vi "HandleMessage.vi"(8 "error in (no error)":errorcluster, 10 "Msg":string, 11 "SHIFTER DATA":T1) -> (0 "error out":errorcluster, 3 "New BP?":bool=TRUE)   [LabVIEW 2013, in "main.lvlib"]
uses:
  main.lvlib
  Components/TypeDef - SHIFTER.ctl
  Components/Dependencies.llb/Exit Event Ref.ctl
  New Design/Controls/Reference Cluster.ctl
  MessageStructure.ctl
  Controls/Enum Variables.ctl
  Controls/Enum Save Action Events.ctl
  Components/Dependencies.llb/TLB_Dependencies.lvlib
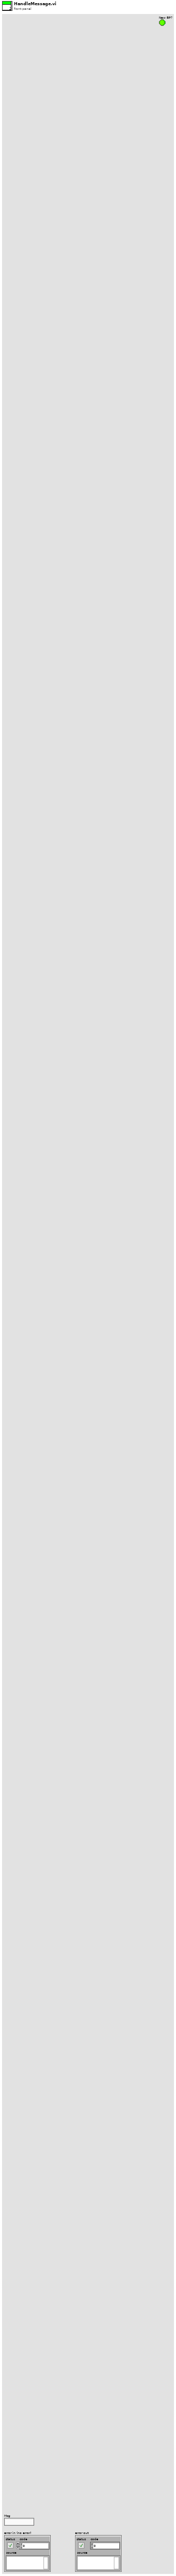
[diagram p1: front panel]
types:
  T1 = typedef "main.lvlib/TypeDef - SHIFTER.ctl" = cluster{"Exit Event":T2, "Terminate Error":errorcluster, "User Parameter Controls":refnum<vi>[], "User Parameters":cluster{"Name":string, "CPR Number":string, "Measuring Type ":string, "Measuring Technique":string, "Measuring Limb":string, "Operator":string, "Doctor":string, "Comment":string, "AdditionalInfo":string, "RightArm":string[][], "LeftArm":string[][], "PalpationRight":string, "PalpationLeft":string, "Puls":dbl, "Temp One":dbl, "Temp Two":dbl, "ActivityBox":bool}, "System Parameters":cluster{"Paper Running?":bool, "GraphSelection":bool, "Date":string, "Active Page":string}, "Data Acquisition":cluster{"Acquisition":bool, "DAQmx Task":refnum<k21>, "DAQmx Error":errorcluster, "Record number":dbl, "RecordPath":path, "AcqDataRef":refnum<vi>, "Duration":timestamp, "Queue":refnum<queue>, "Control?":bool, "RelativeRecordPath":path}, "Reference signal":cluster{"DAQmx  Task ":refnum<k21>, "Monitor":bool, "Events":dbl, "Time":timestamp, "NullEvents":dbl, "RefDataRef":refnum<vi>, "Queue":refnum<queue>}, "Data Process":cluster{"SubpanelRef":refnum<vi>, "ActiveItemTag":string, "Queue":refnum<queue>}, "System Parameter Controls":refnum<vi>[], "Database":cluster{"PatientdataRef":refnum<file>, "PatientdataPath":path, "Blue Pressure":dbl, "Red Pressure":dbl, "ActiveItemTag":string, "Height Adjustment":dbl, "BluePositionArray":dbl[][], "RedPositionArray":dbl[][], "JournalPath":path}, "MWL":cluster{"PatientID":string, "Name":string, "DICOM Info":path, "DICOM Variables":string[], "Worklist":string[][]}, "Control":cluster{"Queue":refnum<queue>, "SignalCluster":cluster{"Pump":bool, "Finger":bool, "Ankle":bool, "Fast Def":bool, "Slow Def":bool, "Init Cal":bool, "Table Pres":bool, "Table":bool}}, "PageMenu":cluster{"VI Reference":refnum<vi>, "Queue":refnum<queue>}, "Profile":cluster{"VI Reference":refnum<vi>, "Queue":refnum<queue>}, "Configuration":cluster{"VI Reference":refnum<vi>, "Queue":refnum<queue>}, "Acquisition":cluster{"VI Reference":refnum<vi>, "Queue":refnum<queue>}, "Data":cluster{"VI Reference":refnum<vi>, "Queue":refnum<queue>}, "Journal":cluster{"VI Reference":refnum<vi>, "Queue":refnum<queue>}, "cRef":T3, "Bluetooth":cluster{"Queue":refnum<queue>, "VI Reference":refnum<vi>}}
  T2 = typedef "main.lvlib/TLB_Dependencies.lvlib/Exit Event Ref.ctl" = refnum<user-event>
  T3 = typedef "main.lvlib/Reference Cluster.ctl" = cluster{"Menu":cluster{"References":cluster{"Stop Acq":refnum<vi>, "MenuExit":refnum<vi>, "MenuStartADC":refnum<vi>, "PersonalInfoString":refnum<vi>, "Profile":refnum<vi>, "Configuration":refnum<vi>, "Acquisition":refnum<vi>, "Data":refnum<vi>, "Journal":refnum<vi>}}, "Profile":cluster{"References":cluster{"Search Patient ID":refnum<vi>, "Name":refnum<vi>, "CommentStr":refnum<vi>, "Listbox Patient ID":refnum<vi>, "ListboxDoctor":refnum<vi>, "ListboxOperator":refnum<vi>, "HospitalName":refnum<vi>, "HospitalDepartment":refnum<vi>, "HospitalAddress":refnum<vi>, "EditHospInfo":refnum<vi>, "Add Patient ID Btn":refnum<vi>, "Query Worklist":refnum<vi>}}, "Configuration":cluster{"References":cluster{"ListboxMeasurementArea":refnum<vi>, "ListboxMeasurementTechnique":refnum<vi>, "ListboxMeasurementMeth":refnum<vi>, "ListboxRightSegmentNr":refnum<vi>, "ListboxLeftSegmentNr":refnum<vi>, "HeightAdjustmentInt":refnum<vi>, "PalpationRight":refnum<vi>, "PalpationLeft":refnum<vi>, "ActivityBox":refnum<vi>}, "New method":cluster{"AddNewMeasurementBtn":refnum<vi>, "Left Time Table":refnum<vi>, "Right Time Table":refnum<vi>}, "Old method":cluster{"LeftArmPressureTable":refnum<vi>, "RightArmPressureTable":refnum<vi>, "SaveArmPressureBtn":refnum<vi>, "Puls":refnum<vi>, "TempTwo":refnum<vi>, "TempOne":refnum<vi>}, "Method":string}, "Acquisition":cluster{"References":cluster{"SegmentAcqString":refnum<vi>, "RingActGraph":refnum<vi>}}, "Data":cluster{"References":cluster{"cmString":refnum<vi>, "AdjustedHeight":refnum<vi>, "Menu":refnum<vi>, "Tangent On/Off":refnum<vi>, "FilterControl":refnum<vi>}}, "Journal":cluster{"References":cluster{"ReportSelection":refnum<vi>, "Data":refnum<vi>, "GenerateReport":refnum<vi>, "Menu":refnum<vi>, "Send To PACS":refnum<vi>}}}
  T4 = typedef "main.lvlib/MessageStructure.ctl" = cluster{"Type":i32, "Device type":i32, "Date":string, "Time":string, "Serial Number":string, "Sys":i32, "Dia":i32, "Puls":i32, "MAP":i32, "Code":string}
  T5 = cluster{"Serial Number":string, "Side":string, "Ignore?":bool}
  T6 = typedef "main.lvlib/Enum Save Action Events.ctl" = enum16{"LoadReportPath", "SaveReportPath", "Load Graph Path", "Save Graph Path", "LoadDataPath", "SaveDataPath", "Load Template Path", "Save Template Path", "Load PressureFactor", "Save PressureFactor", "Init", "Load Listbox", "Save Listbox", "LoadHospInfo", "SaveHospInfo", "Load DICOM Activation", "Save DICOM Activation", "LoadDICOMInfoWL", "SaveDICOMInfoWL", "LoadDICOMInfoPACS", "SaveDICOMInfoPACS", "Load ArmCalcMethod", "Save ArmCalcMethod", "LoadItemTags", "SaveItemTags", "LoadDICOMEncoding", "SaveDICOMEncoding", "LoadJournalType", "SaveJournalType", "LoadAcqFilterType", "SaveAcqFilterType", "Load Sequence", "Save Sequence", "Load Acquisition Mode", "Save Acquisition Mode", "Load General Settings", "Save General Settings", "Load Language", "Save Language", "Load Dicom Tags", "Save Dicom Tags", "Load BT Serial", "Save BT Serial", "Load BT License", "Save BT License"}
  T7 = typedef "main.lvlib/Enum Variables.ctl" = enum16{"SetAcqFilter", "GetAcqFilter", "Set Filter", "Get Filter", "Set Height", "Get Height", "Set Recorded Height", "Get Recorded Height", "Set Blue Pressure", "Get Blue Pressure", "Set Red Pressure", "Get Red Pressure", "Init", "Reset Pressure", "Set Red Cursors", "Get Red Cursors", "Set Blue Cursors", "Get Blue Cursors", "Set Language", "Get Language", "Set Active Graphs", "Get ActiveGraphs", "Set Method", "Get Method", "Set Encryption", "Get Encryption", "Set ExcelVersion", "Get ExcelVersion", "Set DICOM Avail", "Get DICOM Avail", "Set DICOM Encode", "Get DICOM Encode", "Set JournalExport", "Get JournalExport", "Set Sequence", "Get Sequence", "Set DAQ Connected", "Get DAQ Connected", "Set Current Graph", "Get Current Graph", "Set General Settings", "Get Hyphenation", "Set Arm Calc Method", "Get Arm Calc Method", "Set Dicom Tags", "Get Dicom Tags", "Set BT Serial", "Get BT Serial", "Set BT Accepted Serials", "Get BT Accepted Serials", "Get BT License", "Set BT License"}
  T8 = cluster{"Serial Number":string, "Side":string, "Ignore?":bool}[]
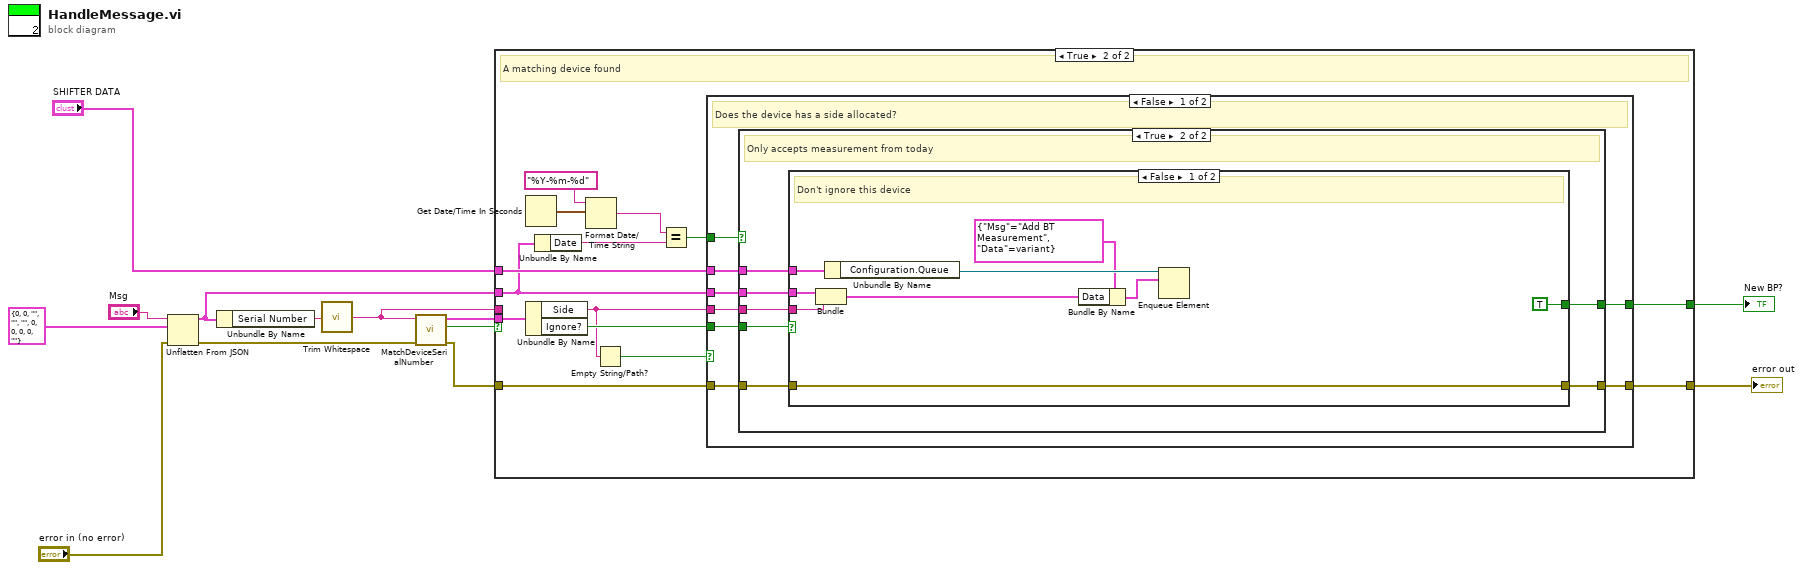
[diagram p0: block diagram]
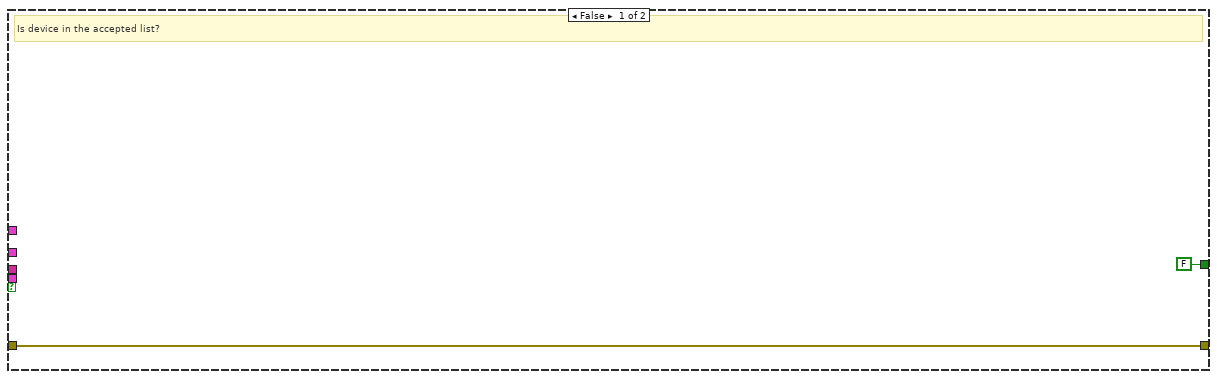
[diagram p2: hidden frame]
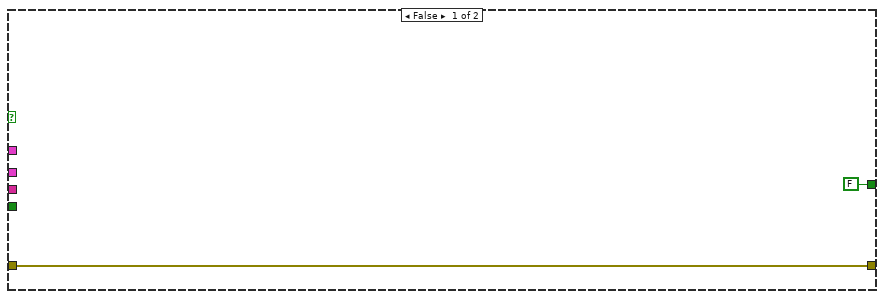
[diagram p3: hidden frame]
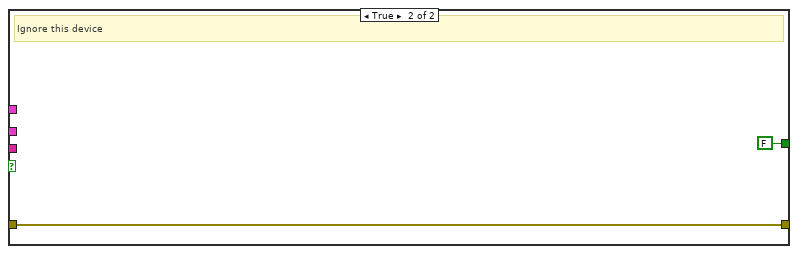
[diagram p4: hidden frame]
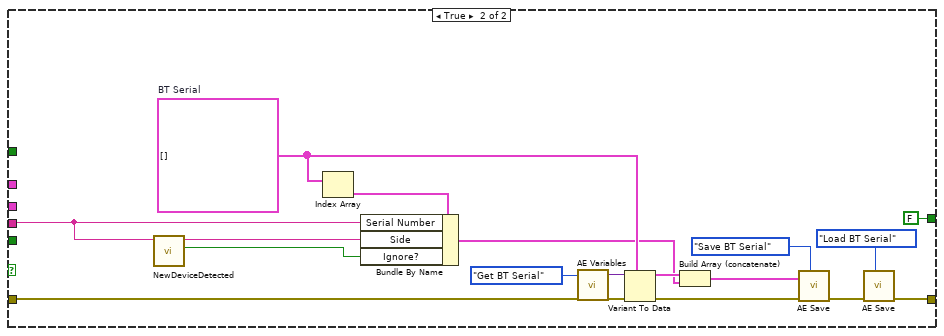
[diagram p5: hidden frame]
diagram:
  n1 = Unflatten From JSON(JSON string="Msg", type and defaults=T4 {"Type"=0, "Device type"=0, "Date"="", "Time"="", "Serial Number"="", "Sys"=0, "Dia"=0, "Puls"=0, "MAP"=0, "Code"=""}, error in (no error)="error in (no error)") -> (value=w7:T4, error out=w10:errorcluster)  [unwired: 4 in]
  n2 = Unbundle By Name(w7) -> ("Serial Number"=w2:string)
  n3 = call <vilib>:"Trim Whitespace.vi"("string"=w2) -> ("trimmed string"=w1:string)  [unwired: 1 in]
  n4 = call "MatchDeviceSerialNumber.vi"("error in (no error)"=w10, "Serial Number"=w1) -> ("error out"=w5:errorcluster, "Match"=w9:bool, "BT Serial"=w8:T5)  [unwired: 7 in]
  n5 = case shown="True" w9 {
    tunnel: w8 -> [_ w29]
    tunnel: w7 -> [_ w23]
    tunnel: "SHIFTER DATA" -> [_ w27]
    tunnel: w5 -> [w15 w26]
    tunnel: [w15 w25] -> w4
    tunnel: w1 -> [_ _]
    tunnel: [FALSE w24] -> w3
    frame False {
      # "Is device in the accepted list?"
    }
    frame True {
      # "A matching device found"
      n6 = Get Date/Time In Seconds() -> (seconds since 1Jan1904=w22:timestamp)
      n7 = Unbundle By Name(w29) -> ("Side"=w17:string, "Ignore?"=w28:bool)
      n8 = Unbundle By Name(w23) -> ("Date"=w19:string)
      n9 = Format Date/Time String(time format string (%c)="%Y-%m-%d", seconds (now)=w22) -> (date/time string=w20:string)  [unwired: 1 in]
      n10 = Empty String/Path?(string/path=w17) -> (empty?=w16:bool)
      n11 = Equal?(x=w20, y=w19) -> (x = y?=w18:bool)
      n12 = case shown="False" w16 {
        tunnel: w28 -> [w37 _]
        tunnel: w27 -> [w36 _]
        tunnel: w26 -> [w35 w61]
        tunnel: [w34 w59] -> w25
        tunnel: [w33 FALSE] -> w24
        tunnel: w23 -> [w32 _]
        tunnel: w18 -> [w31 _]
        tunnel: w17 -> [w30 w60]
        frame False {
          # "Does the device has a side allocated?"
          n13 = case shown="True" w31 {
            tunnel: w37 -> [_ w46]
            tunnel: w30 -> [_ w45]
            tunnel: w36 -> [_ w44]
            tunnel: w35 -> [w39 w43]
            tunnel: [w39 w42] -> w34
            tunnel: [FALSE w41] -> w33
            tunnel: w32 -> [_ w40]
            frame False {
            }
            frame True {
              # "Only accepts measurement from today"
              n14 = case shown="False" w46 {
                tunnel: w45 -> [w52 _]
                tunnel: w40 -> [w53 _]
                tunnel: w44 -> [w51 _]
                tunnel: w43 -> [w55 w57]
                tunnel: [w55 w57] -> w42
                tunnel: [TRUE FALSE] -> w41
                frame False {
                  # "Don't ignore this device"
                  n15 = Bundle(w53, "Side"=w52) -> (w48:cluster{T4, "Side":string})  [unwired: 1 in]
                  n16 = Unbundle By Name(w51) -> ("Configuration.Queue"=w50:refnum<queue>)
                  n17 = Bundle By Name(cluster=cluster{"Msg":string, "Data":variant} {"Msg"="Add BT Measurement", "Data"=variant} ("element"), "Data"=w48) -> (w47:cluster{"Msg":string, "Data":variant})
                  n18 = Enqueue Element(queue=w50, element=w47) -> ()  [unwired: 2 in, 3 out]
                }
                frame True {
                  # "Ignore this device"
                }
              }
            }
          }
        }
        frame True {
          w68 = T8 []  # BT Serial
          n19 = call "NewDeviceDetected.vi"("Serial Number"=w60) -> ("Ignore?"=w62:bool, "Selected Side"=w63:string)  [unwired: 8 in]
          n20 = Index Array(array=w68) -> (element=w67:T5)  [unwired: 1 in]
          n21 = Bundle By Name(cluster=w67, "Serial Number"=w60, "Side"=w63, "Ignore?"=w62) -> (w66:T5)
          n22 = call "AE Variables.vi"("error in (no error)"=w61, "Action"=Enum_Variables."Get BT Serial") -> ("Variant"=w74:variant, "error out"=w70:errorcluster)  [unwired: 10 in, 6 out]
          n23 = Variant To Data(error in=w70, type=w68, Variant=w74) -> (data=w73:T8, error out=w69:errorcluster)
          n24 = Build Array (concatenate)(w73, w66) -> (w72:T8)
          n25 = call "AE Save.vi"("error in (no error)"=w69, "Variant In"=w72, "Action"=Enum_Save_Action_Events."Save BT Serial") -> ("error out"=w64:errorcluster)  [unwired: 6 in, 1 out]
          n26 = call "AE Save.vi"("error in (no error)"=w64, "Action"=Enum_Save_Action_Events."Load BT Serial") -> ("error out"=w59:errorcluster)  [unwired: 7 in, 1 out]
        }
      }
    }
  }
  "error out" <- w4
  "New BP?" <- w3
